vi "Get System Instrument List.vi"(8 "error in (no error)":errorcluster, 10 "Methods Enum":variant) -> (0 "error out":errorcluster, 2 "Instrument List":variant)   [LabVIEW 2020, in "jki_python_bridge.lvlib" / "Server.lvclass"]
uses:
  Server.lvclass
  Server.lvclass/Server.ctl
  <userlib>/_OpenG.lib/lvdata/lvdata.llb/openg_variant.lvlib
  <userlib>/_OpenG.lib/array/array.llb/openg_array.lvlib
  <userlib>/_OpenG.lib/array/array.llb/Remove Duplicates from 1D Array (String)__ogtk.vi
  <userlib>/_OpenG.lib/array/array.llb/Conditional Auto-Indexing Tunnel (String)__ogtk.vi
  <userlib>/_OpenG.lib/array/array.llb/Filter 1D Array with Scalar (String)__ogtk.vi
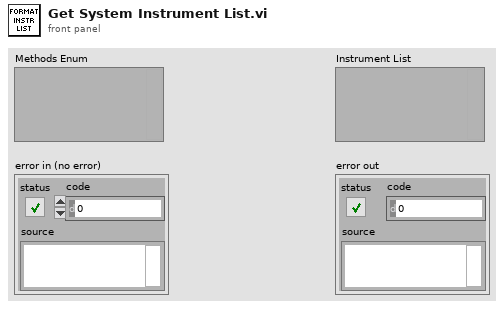
[diagram p1: front panel]
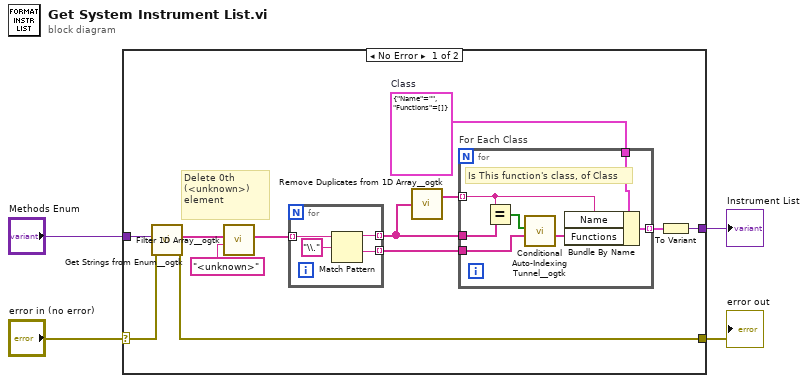
[diagram p0: block diagram]
diagram:
  n1 = case shown="No Error" "error in (no error)" {
    selector: "error in (no error)" -> [w8 w28]
    tunnel: [w16 _] -> w4
    tunnel: [w15 w28] -> w3
    tunnel: "Methods Enum" -> [w14 _]
    frame No Error {
      w13 = cluster{"Name":string, "Functions":string[]} {"Name"="", "Functions"=[]}  # Class
      # "Delete 0th (<unknown>) element"
      n2 = call <userlib>:"Get Strings from Enum__ogtk.vi"("error in (no error)"=w8, "Enum"=w14) -> ("error out"=w15:errorcluster, "Enum Strings"=w6:string[])  [unwired: 8 out]
      n3 = call-poly <userlib>:"Filter 1D Array__ogtk.vi"("items to filter"="<unknown>" ("y"), "array"=w6) -> ("filtered array"=w5:string[])  [unwired: 4 in, 1 out]
      n4 = for {
        tunnel: w5 -> [w27] mode=indexing
        tunnel: [w25] -> w10 mode=indexing
        tunnel: [w24] -> w11 mode=indexing
        n5 = Match Pattern(string=w27, regular expression="\\.") -> (before substring=w25:string, after substring=w24:string)  [unwired: 3 out]
      }
      n6 = call-poly <userlib>:"Remove Duplicates from 1D Array__ogtk.vi"("Input Array"=w10) -> ("Output Array"=w9:string[])  [unwired: 1 out]
      n7 = for "For Each Class" {
        tunnel: w9 -> [w20] mode=indexing
        tunnel: w10 -> [w22]
        tunnel: w11 -> [w18]
        tunnel: [w19] -> w12 mode=indexing
        tunnel: w13 -> [w17]
        # "Is This function's class, of Class"
        n8 = Equal?(x=w20, y=w22) -> (x = y?=w23:bool[])
        n9 = call-poly <userlib>:"Conditional Auto-Indexing Tunnel__ogtk.vi"("Array in"=w18, "Elements to keep"=w23) -> ("Filtered Array out"=w21:string[])  [unwired: 5 out]
        n10 = Bundle By Name(cluster=w17, "Name"=w20, "Functions"=w21) -> (w19:cluster{"Name":string, "Functions":string[]})
      }
      n11 = To Variant(anything=w12) -> (Variant=w16:variant)
    }
    frame Error {
    }
  }
  "Instrument List" <- w4
  "error out" <- w3
